vi "ReversedEngineering CreateStateNodes.vi"(1 "GraphRefToAddNodesTo":refnum<class "Graph.lvclass">=refnum, 2 "StateDiagramReverseOptions":T1={"Clear All Current States"=TRUE, "UseMenuItem"=TRUE, "InsertArrayQueuedElementsVI"="", "Add Actions"=FALSE, "StateDiagramSerachActions"={"Action"=enum."NotTheseVIs", "VINames"=[], "LimitActions(VIs)"=10}, "AddCaseCommentsAsActions"=FALSE, "IgnoreStatesNotUsed"=FALSE, "CommentsSerachActions"={"MinimumTextLength"=0, "OnlyTopLeftComment"=FALSE, "CommentPrefix"=""}, "TransitionMode"=enum."Add to current transtion text", "ActionMode"=enum."Add to current action text"}, 3 "States":T5[](array[typedef])=[{"State"="<<InitialState>>", "TransitionStates"=["\"Init\""], "Actions"=[], "Comments"=[], "TransactionText"=[]}, {"State"=" \"Init\" ", "TransitionStates"=["\"Exit\"", "\"A\"", "\"B\"", "\"1\""], "Actions"=[], "Comments"=[], "TransactionText"=[]}, {"State"=" \"\", \"Idle\" ", "TransitionStates"=["\"C\"", "\"\""], "Actions"=[], "Comments"=[], "TransactionText"=[]}, {"State"=" \"1\" ", "TransitionStates"=["\"2\""], "Actions"=[], "Comments"=[], "TransactionText"=[]}, {"State"=" \"A\" ", "TransitionStates"=[], "Actions"=[], "Comments"=[], "TransactionText"=[]}, {"State"=" \"B\" ", "TransitionStates"=["\"3\""], "Actions"=[], "Comments"=[], "TransactionText"=[]}, {"State"=" \"C\" ", "TransitionStates"=[], "Actions"=[], "Comments"=[], "TransactionText"=[]}, {"State"=" \"2\" ", "TransitionStates"=["\"B\"", "\"3\""], "Actions"=[], "Comments"=[], "TransactionText"=[]}, {"State"=" \"3\" ", "TransitionStates"=["\"B\"", "\"Exit\"", "<<FinalState>>"], "Actions"=[], "Comments"=[], "TransactionText"=[]}, {"State"=" \"Error\" ", "TransitionStates"=["<<FinalState>>"], "Actions"=[], "Comments"=[], "TransactionText"=[]}, {"State"=" \"Exit\" ", "TransitionStates"=["\"Idle\"", "<<FinalState>>"], "Actions"=[], "Comments"=[], "TransactionText"=[]}], 5 "error in (no error)":errorcluster, 7 "graphics":refnum<class "Graphics.lvclass">=refnum, 9 "grid":refnum<class "Grid.lvclass">=refnum) -> (19 "error out":errorcluster)   [LabVIEW 2012]
uses:
  <resource>/Framework/Providers/Open_GDS/UML/ReversedEngineering/ReversedEngineering StateMachineStateInfo.ctl
  <resource>/Framework/Providers/Open_GDS/UML/Graph_class/Graph.lvclass
  <resource>/Framework/Providers/Open_GDS/UML/StateDiagramGraph_class/StateDiagramGraph.lvclass
  <resource>/Framework/Providers/Open_GDS/UML/Graphics_class/Graphics.lvclass
  <resource>/Framework/Providers/Open_GDS/UML/Grid_class/Grid.lvclass
  <resource>/Framework/Providers/Open_GDS/UML/ReversedEngineering/private/ReversedEngineering StateDiagramReverseOptions.ctl
  <resource>/Framework/Providers/Open_GDS/UML/ReversedEngineering/private/ReversedEngineering StateDiagramSerachActions.ctl
  <resource>/Framework/Providers/Open_GDS/UML/ReversedEngineering/ReversedEngineering StateAnalyseVIAction.ctl
  <resource>/Framework/Providers/Open_GDS/UML/ReversedEngineering/private/ReversedEngineering StateDiagramCommentSearchType.ctl
  <resource>/Framework/Providers/Open_GDS/UML/AbstractNode_class/AbstractNode.lvclass
  <resource>/Framework/Providers/Open_GDS/UML/StateNode_class/StateNode.lvclass
  <resource>/Framework/Providers/Open_GDS/UML/MultiLineString_class/MultiLineString.lvclass
  <resource>/Framework/Providers/Open_GDS/UML/StateReverse_class/StateReverse.lvclass
  <resource>/Framework/Providers/Open_GDS/UML/General/Point/Point Point2D.ctl
  <resource>/Framework/Providers/Open_GDS/UML/RectangularNode_class/RectangularNode.lvclass
  <resource>/Framework/Providers/Open_GDS/UML/General/Rectangle/Rectangle DirectionToTest.ctl
  <resource>/Framework/Providers/Open_GDS/UML/General/Rectangle/Rectangle Rectangle2D.ctl
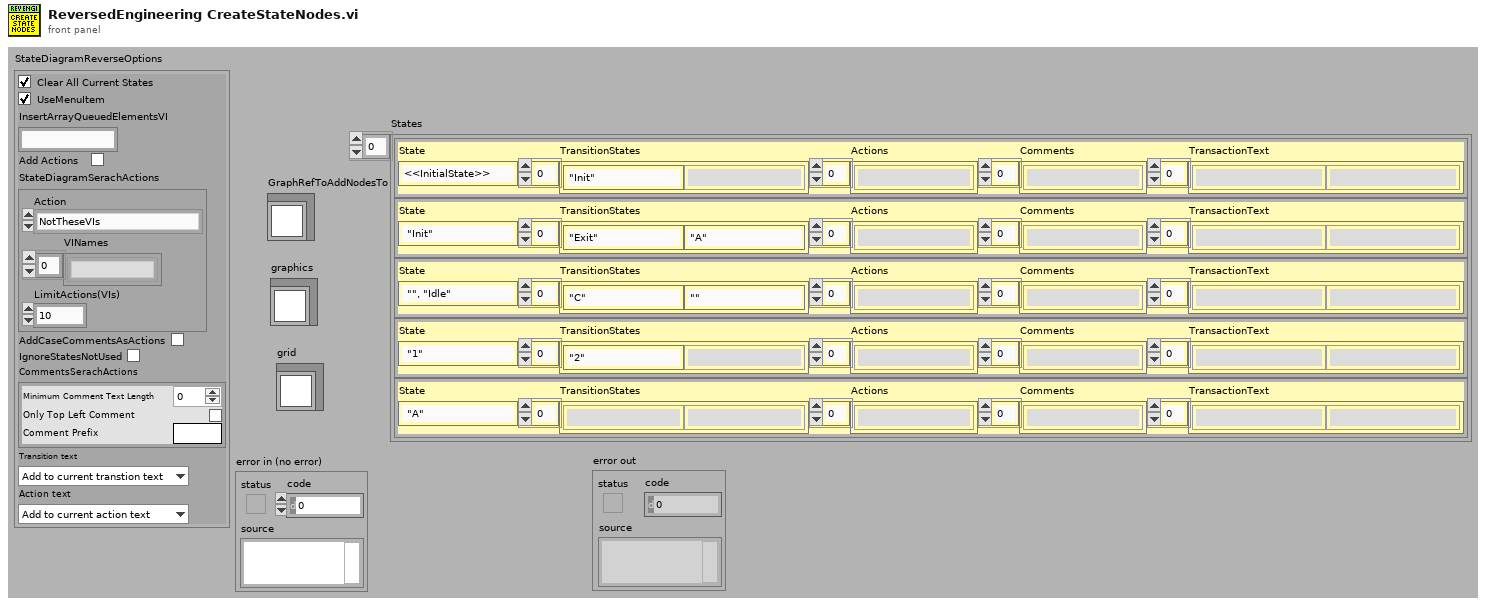
[diagram p1: front panel]
types:
  T1 = typedef "ReversedEngineering StateDiagramReverseOptions.ctl" = cluster{"Clear All Current States":bool, "UseMenuItem":bool, "InsertArrayQueuedElementsVI":string, "Add Actions":bool, "StateDiagramSerachActions":T2, "AddCaseCommentsAsActions":bool, "IgnoreStatesNotUsed":bool, "CommentsSerachActions":T4, "TransitionMode":enum16{"Add to current transtion text", "Replace transition text"}, "ActionMode":enum16{"Add to current action text", "Replace action text"}}
  T2 = typedef "ReversedEngineering StateDiagramSerachActions.ctl" = cluster{"Action":T3, "VINames":string[], "LimitActions(VIs)":i32}
  T3 = typedef "ReversedEngineering StateAnalyseVIAction.ctl" = enum16{"OnlyTheseVIs", "NotTheseVIs"}
  T4 = typedef "ReversedEngineering StateDiagramCommentSearchType.ctl" = cluster{"MinimumTextLength":i32, "OnlyTopLeftComment":bool, "CommentPrefix":string}
  T5 = typedef "ReversedEngineering StateMachineStateInfo.ctl" = cluster{"State":string, "TransitionStates":string[], "Actions":string[], "Comments":string[], "TransactionText":string[]}
  T6 = enum16{"Add to current action text", "Replace action text"}
  T7 = typedef "Point Point2D.ctl" = cluster{"x":dbl, "y":dbl}
  T8 = typedef "Rectangle Rectangle2D.ctl" = cluster{"x":dbl, "y":dbl, "width":dbl, "height":dbl}
  T9 = typedef "Rectangle DirectionToTest.ctl" = enum16{"E-S-W-N", "ES-S-WS"}
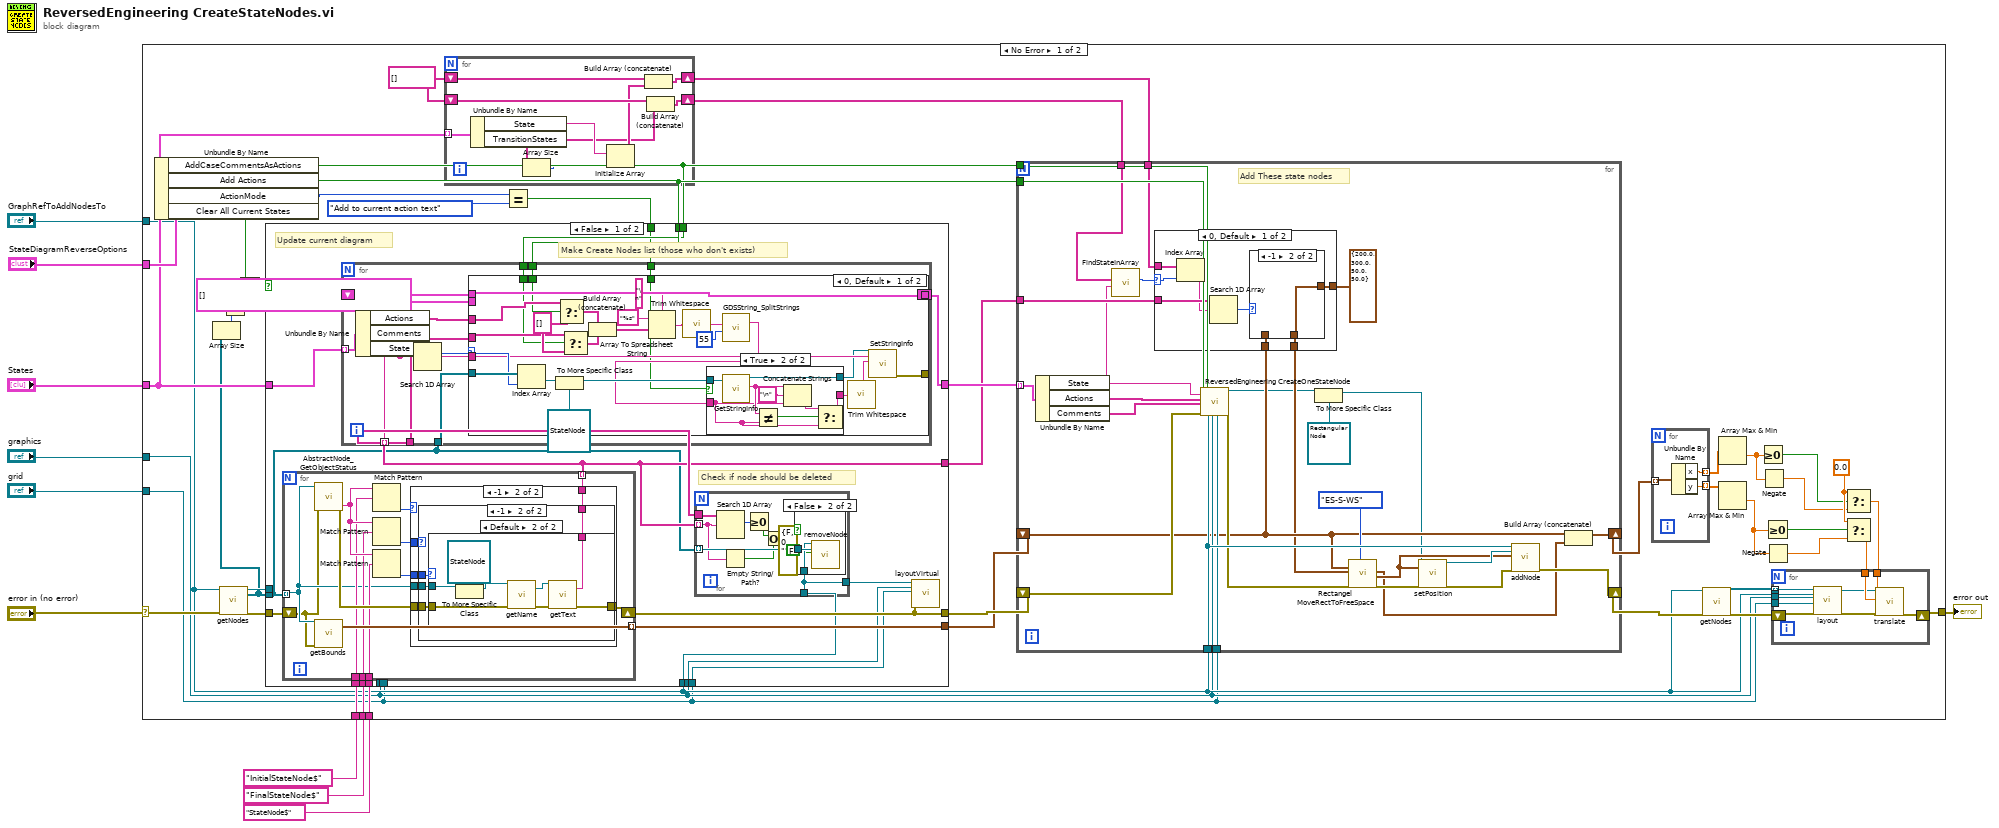
[diagram p0: block diagram]
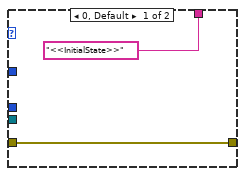
[diagram p3: hidden frame]
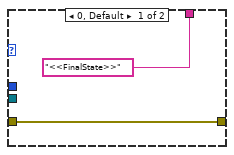
[diagram p4: hidden frame]
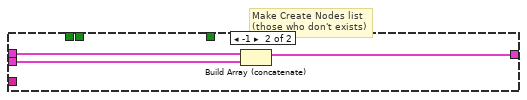
[diagram p7: hidden frame]
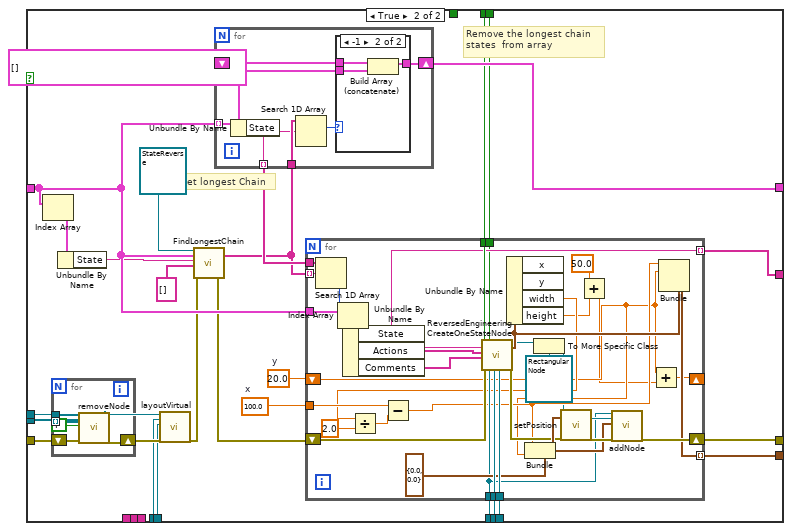
[diagram p8: hidden frame]
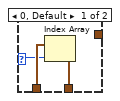
[diagram p10: hidden frame]
diagram:
  n1 = case shown="No Error" "error in (no error)" {
    selector: "error in (no error)" -> [w53 w314]
    tunnel: [w39 w314] -> w9
    tunnel: "States" -> [w30 _]
    tunnel: "GraphRefToAddNodesTo" -> [w17 _]
    tunnel: "graphics" -> [w16 _]
    tunnel: "grid" -> [w15 _]
    tunnel: "StateDiagramReverseOptions" -> [w34 _]
    tunnel: "InitialStateNode$" -> [w26 _]
    tunnel: "FinalStateNode$" -> [w25 _]
    tunnel: "StateNode$" -> [w24 _]
    frame No Error {
      w29 = string[] []
      w48 = 0.0 ("t")
      n2 = Unbundle By Name(w34) -> ("AddCaseCommentsAsActions"=w14:bool, "Add Actions"=w31:bool, "ActionMode"=w13:T6, "Clear All Current States"=w21:bool)
      n3 = call-dynamic "getNodes.vi"("reference"=w17, "error in (no error)"=w53) -> ("reference out"=w33:refnum<class "Graph.lvclass">, "nodes"=w23:refnum<class "AbstractNode.lvclass">[], "error out"=w37:errorcluster)  [unwired: 15 in]
      n4 = Array Size(array=w23) -> (size(s)=w20:i32)
      n5 = Equal To 0?(x=w20) -> (x = 0?=w19:bool)
      n6 = Or(x=w21, y=w19) -> (x .or. y?=w22:bool)
      n7 = for {
        tunnel: w30 -> [w62] mode=indexing
        shift-right: [w57] -> w28
        shift-left: w29 -> [w59]
        shift-right: [w56] -> w18
        shift-left: w29 -> [w58]
        n8 = Unbundle By Name(w62) -> ("State"=w60:string, "TransitionStates"=w54:string[])
        n9 = Array Size(array=w54) -> (size(s)=w61:i32)
        n10 = Initialize Array(w60, w61) -> (w55:string[])
        n11 = Build Array (concatenate)(w59, w55) -> (w57:string[])
        n12 = Build Array (concatenate)(w58, w54) -> (w56:string[])
      }
      n13 = Equal?(x=w13, y=T6."Add to current action text") -> (x = y?=w11:bool)
      n14 = case shown="False" w22 {
        tunnel: w30 -> [w81 w188]
        tunnel: w23 -> [w71 w208]
        tunnel: w37 -> [w80 w207]
        tunnel: [w70 w201] -> w36
        tunnel: [w79 w197] -> w35
        tunnel: w33 -> [_ w192]
        tunnel: [w77 w204] -> w32
        tunnel: w31 -> [w65 w202]
        tunnel: w17 -> [w69 w200]
        tunnel: w16 -> [w67 w199]
        tunnel: w15 -> [w66 w198]
        tunnel: [w72 w194] -> w27
        tunnel: w26 -> [w76 _]
        tunnel: w25 -> [w75 _]
        tunnel: w24 -> [w74 _]
        tunnel: w16 -> [_ w191]
        tunnel: w15 -> [_ w190]
        tunnel: w14 -> [w64 w182]
        tunnel: w11 -> [w63 _]
        frame False {
          # "Check if node should be deleted"
          # "Make Create Nodes list (those who don't exists)"
          # "Update current diagram"
          n15 = for {
            tunnel: w71 -> [w97] mode=indexing
            shift-right: [w94] -> w70
            shift-left: w80 -> [w96]
            tunnel: [w106] -> w79 mode=indexing
            tunnel: [w95] -> w72 mode=indexing
            tunnel: w76 -> [w100]
            tunnel: w75 -> [w99]
            tunnel: w74 -> [w98]
            n16 = call <resource>:"AbstractNode_GetObjectStatus.vi"("reference in"=w97, "error in (no error)"=w96) -> ("Class name"=w103:string, "error out"=w101:errorcluster)  [unwired: 16 out]
            n17 = call-dynamic "getBounds.vi"("reference"=w97, "error in (no error)"=w96) -> ("bounds"=w106:T8)  [unwired: 15 in, 2 out]
            n18 = Match Pattern(string=w103, regular expression=w100) -> (offset past match=w104:i32)  [unwired: 4 out]
            n19 = Match Pattern(string=w103, regular expression=w99) -> (offset past match=w105:i32)  [unwired: 4 out]
            n20 = Match Pattern(string=w103, regular expression=w98) -> (offset past match=w102:i32)  [unwired: 4 out]
            n21 = case shown="-1" w104 {
              tunnel: w101 -> [w107 w114]
              tunnel: w102 -> [_ w113]
              tunnel: [w107 w112] -> w94
              tunnel: ["<<InitialState>>" ("text") w111] -> w95
              tunnel: w97 -> [_ w110]
              tunnel: w105 -> [_ w109]
              frame 0, Default {
              }
              frame -1 {
                n22 = case shown="-1" w109 {
                  tunnel: w114 -> [w115 w121]
                  tunnel: w113 -> [_ w120]
                  tunnel: [w115 w119] -> w112
                  tunnel: ["<<FinalState>>" ("text") w118] -> w111
                  tunnel: w110 -> [_ w117]
                  frame 0, Default {
                  }
                  frame -1 {
                    n23 = case shown="Default" w120 {
                      tunnel: w117 -> [_ w124]
                      tunnel: w121 -> [w122 w130]
                      tunnel: [w122 w127] -> w119
                      tunnel: [_ w126] -> w118
                      frame -1 {
                      }
                      frame Default {
                        n24 = To More Specific Class(target class=refnum<class "StateNode.lvclass"> refnum ("reference"), reference=w124) -> (specific class reference=w123:refnum<class "StateNode.lvclass">)  [unwired: 1 in, 1 out]
                        n25 = call-dynamic "getName.vi"("reference"=w123, "error in (no error)"=w130) -> ("name"=w129:refnum<class "MultiLineString.lvclass">, "error out"=w128:errorcluster)  [unwired: 15 in, 1 out]
                        n26 = call-dynamic "getText.vi"("reference"=w129, "error in (no error)"=w128) -> ("text"=w126:string, "error out"=w127:errorcluster)  [unwired: 15 in, 1 out]
                      }
                    }
                  }
                }
              }
            }
          }
          n27 = for {
            tunnel: w81 -> [w137] mode=indexing
            shift-right: [w141] -> w77
            shift-left: T5[] [] -> [w142]
            tunnel: w72 -> [w140]
            tunnel: w71 -> [w138]
            tunnel: [w135] -> w73 mode=indexing
            tunnel: w65 -> [w133]
            tunnel: w64 -> [w132]
            tunnel: w63 -> [w131]
            n28 = Unbundle By Name(w137) -> ("Actions"=w134:string[], "Comments"=w136:string[], "State"=w135:string)
            n29 = Search 1D Array(1D array=w140, element=w135) -> (index of element=w139:i32)  [unwired: 1 out]
            n30 = case shown="0, Default" w139 {
              selector: w139 -> [w166 _]
              tunnel: w142 -> [w168 w181]
              tunnel: [w168 w180] -> w141
              tunnel: w137 -> [_ w179]
              tunnel: w138 -> [w167 _]
              tunnel: w136 -> [w157 _]
              tunnel: w135 -> [w165 _]
              tunnel: [w162 _] -> _
              tunnel: w134 -> [w159 _]
              tunnel: w133 -> [w156 _]
              tunnel: w132 -> [w155 _]
              tunnel: w131 -> [w144 _]
              frame 0, Default {
                w158 = string[] [] ("f")
                n31 = Index Array(array=w167, index=w166) -> (element=w163:refnum<class "AbstractNode.lvclass">)
                n32 = To More Specific Class(target class=refnum<class "StateNode.lvclass"> refnum ("reference"), reference=w163) -> (specific class reference=w148:refnum<class "StateNode.lvclass">)  [unwired: 1 in, 1 out]
                n33 = Select(t=w159, s=w156, f=w158) -> (s? t:f=w161:string[])
                n34 = Select(t=w157, s=w155, f=w158) -> (s? t:f=w160:string[])
                n35 = Build Array (concatenate)(w161, w160) -> (w149:string[])
                n36 = Array To Spreadsheet String(delimiter (Tab)="\n", array=w149, 3:"%s" ("format string")) -> (spreadsheet string=w154:string)
                n37 = call <vilib>:"Trim Whitespace.vi"("string"=w154) -> ("trimmed string"=w151:string)  [unwired: 1 in]
                n38 = call <resource>:"GDSString_SplitStrings.vi"("MaxCharactersPerRow(25)"=55, "StringIn"=w151) -> ("String Out"=w145:string)  [unwired: 9 in]
                n39 = case shown="True" w144 {
                  tunnel: w148 -> [w169 w178]
                  tunnel: [w169 w177] -> w147
                  tunnel: [w170 w171] -> w146
                  tunnel: w145 -> [w170 w173]
                  frame False {
                  }
                  frame True {
                    n40 = call-dynamic "GetStringInfo.vi"("reference in"=w178) -> ("reference out"=w177:refnum<class "StateNode.lvclass">, "Action"=w175:string)  [unwired: 15 in, 2 out]
                    n41 = Not Equal?(x=w175, y=w173) -> (x != y?=w174:bool)
                    n42 = Concatenate Strings(w175, "\n" ("string"), w173) -> (w172:string)
                    n43 = Select(t=w172, s=w174, f=w173) -> (s? t:f=w171:string)
                  }
                }
                n44 = call <vilib>:"Trim Whitespace.vi"("string"=w146) -> ("trimmed string"=w143:string)  [unwired: 1 in]
                n45 = call <resource>:"SetStringInfo.vi"("reference"=w147, "State"=w165, "Action"=w143) -> ("error out"=w162:errorcluster)  [unwired: 1 in, 15 out]
              }
              frame -1 {
                # "Make Create Nodes list (those who don't exists)"
                n46 = Build Array (concatenate)(w181, w179) -> (w180:T5[])
              }
            }
          }
          n47 = for {
            tunnel: w73 -> [w89]
            tunnel: w72 -> [w85] mode=indexing
            tunnel: w71 -> [w88] mode=indexing
            tunnel: w69 -> [w87]
            tunnel: [w87] -> w68
            n48 = Search 1D Array(1D array=w89, element=w85) -> (index of element=w86:i32)  [unwired: 1 out]
            n49 = Empty String/Path?(string/path=w85) -> (empty?=w83:bool)
            n50 = Greater Or Equal To 0?(x=w86) -> (x >= 0?=w84:bool)
            n51 = Or(x=w84, y=w83) -> (x .or. y?=w82:bool)
            n52 = case shown="False" w82 {
              tunnel: w88 -> [_ w93]
              tunnel: w87 -> [_ w92]
              frame True {
              }
              frame False {
                n53 = call-dynamic "removeNode.vi"("reference"=w92, "node"=w93, "RemoveChildrenIfAny(False)"=FALSE, "error in (no error)"=errorcluster {"status"=FALSE, "code"=0, "source"=""}) -> ()  [unwired: 14 in, 2 out]
              }
            }
          }
          n54 = call <resource>:"layoutVirtual.vi"("reference"=w68, "graphics"=w67, "grid"=w66, "error in (no error)"=w70) -> ()  [unwired: 16 out]
        }
        frame True {
          w195 = 20.0  # y
          w196 = 100.0  # x
          # "Remove the longest chain\nstates  from array"
          # "Get longest Chain"
          n55 = Index Array(array=w188) -> (element=w206:T5)  [unwired: 1 in]
          n56 = for {
            tunnel: w192 -> [w258]
            tunnel: w208 -> [w257] mode=indexing
            shift-right: [w256] -> w193
            shift-left: w207 -> [w255]
            n57 = call-dynamic "removeNode.vi"("reference"=w258, "node"=w257, "RemoveChildrenIfAny(False)"=FALSE, "error in (no error)"=w255) -> ("error out"=w256:errorcluster)  [unwired: 14 in, 1 out]
          }
          n58 = Unbundle By Name(w206) -> ("State"=w187:string)
          n59 = call <resource>:"layoutVirtual.vi"("reference"=w192, "graphics"=w191, "grid"=w190, "error in (no error)"=w193) -> ("error out"=w184:errorcluster)  [unwired: 15 out]
          n60 = call-dynamic "FindLongestChain.vi"("object in"=refnum<class "StateReverse.lvclass"> refnum, "States"=w188, "State"=w187, "StateSeqencies"=string[] [], "error in (no error)"=w184) -> ("StateSeqenciesOut"=w185:string[], "error out"=w183:errorcluster)  [unwired: 13 in]
          n61 = for {
            tunnel: w188 -> [w247] mode=indexing
            shift-right: [w248] -> w204
            shift-left: T5[] [] -> [w249]
            tunnel: w185 -> [w246]
            tunnel: [w244] -> w203 mode=indexing
            n62 = Unbundle By Name(w247) -> ("State"=w244:string)
            n63 = Search 1D Array(1D array=w246, element=w244) -> (index of element=w245:i32)  [unwired: 1 out]
            n64 = case shown="-1" w245 {
              tunnel: w249 -> [w250 w253]
              tunnel: [w250 w252] -> w248
              tunnel: w247 -> [_ w251]
              frame 0, Default {
              }
              frame -1 {
                n65 = Build Array (concatenate)(w253, w251) -> (w252:T5[])
              }
            }
          }
          n66 = for {
            tunnel: w185 -> [w242] mode=indexing
            tunnel: w203 -> [w243]
            tunnel: w188 -> [w240]
            tunnel: w202 -> [w238]
            shift-right: [w231] -> w201
            shift-left: w183 -> [w236]
            shift-right: [w215] -> _
            shift-left: w195 -> [w219]
            tunnel: w200 -> [w225]
            tunnel: w199 -> [w235]
            tunnel: w198 -> [w234]
            tunnel: [w226] -> w197 mode=indexing
            tunnel: w196 -> [w224]
            tunnel: [w214] -> w194 mode=indexing
            tunnel: w182 -> [w209]
            n67 = Search 1D Array(1D array=w243, element=w242) -> (index of element=w241:i32)  [unwired: 1 out]
            n68 = Index Array(array=w240, index=w241) -> (element=w239:T5)
            n69 = Unbundle By Name(w239) -> ("State"=w214:string, "Actions"=w237:string[], "Comments"=w210:string[])
            n70 = call <resource>:"ReversedEngineering CreateOneStateNode.vi"("Add Actions"=w238, "State"=w214, "Actions"=w237, "Comments"=w210, "error in"=w236, "Add Comments"=w209, "GraphRefToAddNodesTo"=w225, "graphics"=w235, "grid"=w234) -> ("reference out"=w212:refnum<class "AbstractNode.lvclass">, "bounds"=w227:T8, "error out"=w228:errorcluster)  [unwired: 5 in, 3 out]
            n71 = Unbundle By Name(w227) -> ("width"=w223:dbl, "height"=w218:dbl)  [unwired: 2 out]
            n72 = Divide(x=w223, y=2.0) -> (x/y=w221:dbl)
            n73 = Subtract(x=w224, y=w221) -> (x-y=w220:dbl)
            n74 = Bundle(cluster=T7 {"x"=0.0, "y"=0.0} ("point"), "x"=w220, "y"=w219) -> (w229:T7)
            n75 = To More Specific Class(target class=refnum<class "RectangularNode.lvclass"> refnum ("reference"), reference=w212) -> (specific class reference=w211:refnum<class "RectangularNode.lvclass">)  [unwired: 1 in, 1 out]
            n76 = call <resource>:"setPosition.vi"("reference"=w211, "pos"=w229, "error in (no error)"=w228) -> ("reference out"=w233:refnum<class "RectangularNode.lvclass">, "error out"=w232:errorcluster)  [unwired: 2 in, 13 out]
            n77 = Add(x=50.0, y=w218) -> (x+y=w216:dbl)
            n78 = call-dynamic "addNode.vi"("reference"=w225, "node"=w233, "point"=w229, "error in (no error)"=w232) -> ("error out"=w231:errorcluster)  [unwired: 14 in, 1 out]
            n79 = Add(x=w219, y=w216) -> (x+y=w215:dbl)
            n80 = Bundle(cluster=w227, "x"=w220, "y"=w219) -> (w226:T8)  [unwired: 2 out]
          }
        }
      }
      n81 = for {
        shift-right: [w300] -> w40
        shift-left: w36 -> [w292]
        tunnel: w16 -> [w288]
        tunnel: w17 -> [w289]
        shift-right: [w299] -> w52
        shift-left: w35 -> [w282]
        tunnel: w32 -> [w298] mode=indexing
        tunnel: w31 -> [w290]
        tunnel: w15 -> [w287]
        tunnel: w18 -> [w275]
        tunnel: w28 -> [w284]
        tunnel: w27 -> [w283]
        tunnel: w14 -> [w272]
        # "Add These state nodes"
        n82 = Unbundle By Name(w298) -> ("State"=w276:string, "Actions"=w291:string[], "Comments"=w273:string[])
        n83 = call <resource>:"FindStateInArray.vi"("TransactionState"=w276, "AllCaseStates"=w275) -> ("index of element"=w274:i32)  [unwired: 7 in, 2 out]
        n84 = case shown="0, Default" w274 {
          selector: w274 -> [w308 _]
          tunnel: w284 -> [w307 _]
          tunnel: w283 -> [w306 _]
          tunnel: w282 -> [w303 _]
          tunnel: [w302 w313] -> w281
          tunnel: T8 {"x"=200.0, "y"=300.0, "width"=50.0, "height"=50.0} ("bounds") -> [w301 w313]
          frame 0, Default {
            n85 = Index Array(array=w307, index=w308) -> (element=w305:string)
            n86 = Search 1D Array(1D array=w306, element=w305) -> (index of element=w304:i32)  [unwired: 1 in]
            n87 = case shown="-1" w304 {
              selector: w304 -> [w310 _]
              tunnel: w303 -> [w311 _]
              tunnel: [w309 w312] -> w302
              tunnel: w301 -> [_ w312]
              frame 0, Default {
                n88 = Index Array(array=w311, index=w310) -> (element=w309:T8)
              }
              frame -1 {
              }
            }
          }
          frame -1 {
          }
        }
        n89 = call <resource>:"ReversedEngineering CreateOneStateNode.vi"("Add Actions"=w290, "State"=w276, "Actions"=w291, "Comments"=w273, "error in"=w292, "Add Comments"=w272, "GraphRefToAddNodesTo"=w289, "graphics"=w288, "grid"=w287) -> ("reference out"=w279:refnum<class "AbstractNode.lvclass">, "error out"=w286:errorcluster)  [unwired: 5 in, 4 out]
        n90 = To More Specific Class(target class=refnum<class "RectangularNode.lvclass"> refnum ("reference"), reference=w279) -> (specific class reference=w278:refnum<class "RectangularNode.lvclass">)  [unwired: 1 in, 1 out]
        n91 = call <resource>:"Rectangel MoveRectToFreeSpace.vi"("BoundsArray"=w282, "bounds"=w281, "error in (no error)"=w286, "DirectionsToTest(E-S-W-N)"=Rectangle_DirectionToTest."ES-S-WS") -> ("BoundsOut"=w293:T8, "point"=w295:T7, "error out"=w297:errorcluster)  [unwired: 13 out]
        n92 = call <resource>:"setPosition.vi"("reference"=w278, "pos"=w295, "error in (no error)"=w297) -> ("reference out"=w296:refnum<class "RectangularNode.lvclass">, "error out"=w294:errorcluster)  [unwired: 2 in, 13 out]
        n93 = call-dynamic "addNode.vi"("reference"=w289, "node"=w296, "point"=w295, "error in (no error)"=w294) -> ("error out"=w300:errorcluster)  [unwired: 14 in, 1 out]
        n94 = Build Array (concatenate)(w282, w293) -> (w299:T8[])
      }
      n95 = for {
        tunnel: w52 -> [w271] mode=indexing
        tunnel: [w270] -> w51 mode=indexing
        tunnel: [w269] -> w50 mode=indexing
        n96 = Unbundle By Name(w271) -> ("x"=w270:dbl, "y"=w269:dbl)
      }
      n97 = call-dynamic "getNodes.vi"("reference"=w17, "error in (no error)"=w40) -> ("nodes"=w38:refnum<class "AbstractNode.lvclass">[])  [unwired: 15 in, 2 out]
      n98 = Array Max & Min(array=w51) -> (min value=w45:dbl)  [unwired: 3 out]
      n99 = Array Max & Min(array=w50) -> (min value=w43:dbl)  [unwired: 3 out]
      n100 = Greater Or Equal To 0?(x=w45) -> (x >= 0?=w46:bool)
      n101 = Negate(x=w45) -> (-x=w44:dbl)
      n102 = Greater Or Equal To 0?(x=w43) -> (x >= 0?=w42:bool)
      n103 = Negate(x=w43) -> (-x=w41:dbl)
      n104 = Select(t=w48, s=w46, f=w44) -> (s? t:f=w49:dbl)
      n105 = Select(t=w48, s=w42, f=w41) -> (s? t:f=w47:dbl)
      n106 = for {
        tunnel: w49 -> [w268]
        tunnel: w47 -> [w267]
        shift-right: [w266] -> w39
        shift-left: w40 -> [w265]
        tunnel: w38 -> [w262] mode=indexing
        tunnel: w17 -> [w261]
        tunnel: w16 -> [w260]
        tunnel: w15 -> [w259]
        n107 = call-dynamic "layout.vi"("reference"=w262, "graph"=w261, "graphics"=w260, "grid"=w259, "error in (no error)"=w265) -> ("reference out"=w263:refnum<class "AbstractNode.lvclass">, "error out"=w264:errorcluster)  [unwired: 13 in]
        n108 = call-dynamic "translate.vi"("reference"=w263, "dx"=w268, "dy"=w267, "error in (no error)"=w264) -> ("error out"=w266:errorcluster)  [unwired: 14 in, 1 out]
      }
    }
    frame Error {
    }
  }
  "error out" <- w9
